vi "Rotation Matrix to Quaternion.vi"(1 "rotation matrix":T1) -> (0 "quaternion":T2)   [LabVIEW 2017, in "NI_Kinematics.lvlib"]
doc: "Converts a <B>rotation matrix</B> to the corresponding unit quaternion."
uses:
  <vilib>/robotics/Kinematics/NI_Kinematics.lvlib
  <vilib>/robotics/Kinematics/Quaternion.ctl
  <vilib>/Analysis/Matrix/Datatypes/RealMatrix.ctl
  <vilib>/Analysis/Matrix/NI_Matrix.lvlib
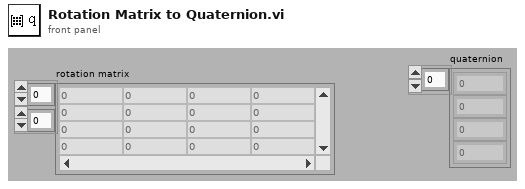
[diagram p1: front panel]
types:
  T1 = typedef "NI_Matrix.lvlib/RealMatrix.ctl" = dbl[][]
  T2 = typedef "NI_Kinematics.lvlib/Quaternion.ctl" = dbl[]
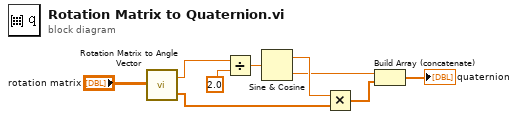
[diagram p0: block diagram]
diagram:
  n1 = call <vilib>:"Rotation Matrix to Angle Vector.vi"("rotation matrix"="rotation matrix") -> ("angle"=w8:dbl, "vector"=w1:dbl[])
  n2 = Divide(x=w8, y=2.0) -> (x/y=w7:dbl)
  n3 = Sine & Cosine(0:w7) -> (1:w5:dbl, 2:w4:dbl)
  n4 = Multiply(x=w5, y=w1) -> (x*y=w3:dbl[])
  n5 = Build Array (concatenate)(w4, w3) -> (→"quaternion":dbl[])
